vi "AddAdditionalFields.vi"(8 "error in (no error)":errorcluster, 10 "Menu":refnum<class "MGI_Menu.lvclass">, 11 "MGI_TrayItem in":refnum<class "MGI_TrayItem.lvclass">) -> (0 "error out":errorcluster, 2 "Menu out":refnum<class "MGI_Menu.lvclass">, 3 "MGI_TrayItem out":refnum<class "MGI_TrayItem.lvclass">)   [LabVIEW 2016, in "MGI_TrayItem.lvclass"]
doc: "Adds shorcut and default item indicators to the menu.\n\nAuthored by Derek E. Trepanier\nsupport@mooregoodideas.com\nwww.mooregoodideas.com\n\nCopyright (c) 2012, Moore Good Ideas, Inc.\n\nAll rights reserved.\n\nRedistribution and use in source and binary forms, with or without modification, are permitted provided that the following conditions are met:\n\n * Redistributions of source code must retain the above copyright notice, this list of conditions and the following disclaimer.\n * Redistributions in binary form must reproduce the above copyright notice, this list of conditions and the following disclaimer in the documentation and/or other materials provided with the distribution.\n * Neither the name of Moore Good Ideas, Inc. nor the names of its contributors may be used to endorse or promote products derived from this software without specific prior written permission.\n\nTHIS SOFTWARE IS PROVIDED BY THE COPYRIGHT HOLDERS AND CONTRIBUTORS \"AS IS\" AND ANY EXPRESS OR IMPLIED WARRANTIES, INCLUDING, BUT NOT LIMITED TO, THE IMPLIED WARRANTIES OF MERCHANTABILITY AND FITNESS FOR A PARTICULAR PURPOSE ARE DISCLAIMED. IN NO EVENT SHALL THE COPYRIGHT OWNER OR CONTRIBUTORS BE LIABLE FOR ANY DIRECT, INDIRECT, INCIDENTAL, SPECIAL, EXEMPLARY, OR CONSEQUENTIAL DAMAGES (INCLUDING, BUT NOT LIMITED TO, PROCUREMENT OF SUBSTITUTE GOODS OR SERVICES; LOSS OF USE, DATA, OR PROFITS; OR BUSINESS INTERRUPTION) HOWEVER CAUSED AND ON ANY THEORY OF LIABILITY, WHETHER IN CONTRACT, STRICT LIABILITY, OR TORT (INCLUDING NEGLIGENCE OR OTHERWISE) ARISING IN ANY WAY OUT OF THE USE OF THIS SOFTWARE, EVEN IF ADVISED OF THE POSSIBILITY OF SUCH DAMAGE."
uses:
  <userlib>/_MGI/Menu Building/MenuItem/TrayIcon/MGI_TrayItem.lvclass
  C:/Program Files (x86)/National Instruments/LabVIEW 2016/user.lib/_MGI/Menu Building/MenuItem/MGI_MenuItem.lvclass
  <userlib>/_MGI/Menu Building/MenuTypes/MGI_Menu.lvclass
  <userlib>/_MGI/Menu Building/MenuTypes/TrayIcon/MGI_TrayIcon.lvclass
  C:/Program Files (x86)/National Instruments/LabVIEW 2016/user.lib/_MGI/Menu Building/MenuTypes/MGI_Menu.lvclass
  <userlib>/_MGI/Menu Building/MenuItem/TrayIcon/MGI_TrayItem.lvclass/MGI_TrayItem.ctl
  System.Windows.Forms
  <userlib>/_MGI/Menu Building/MenuItem/Read Full Tag.vi
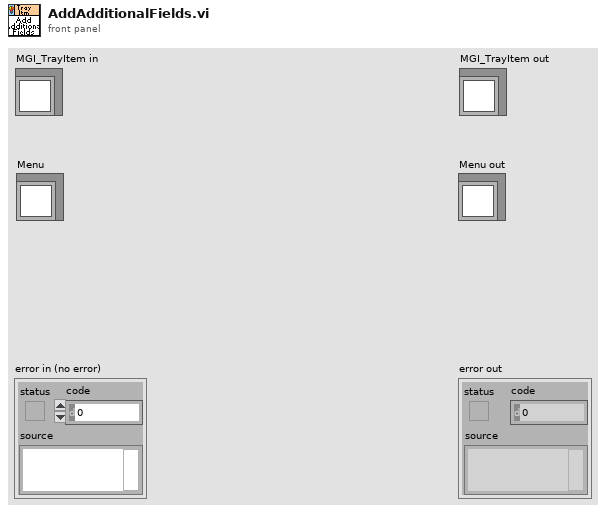
[diagram p1: front panel]
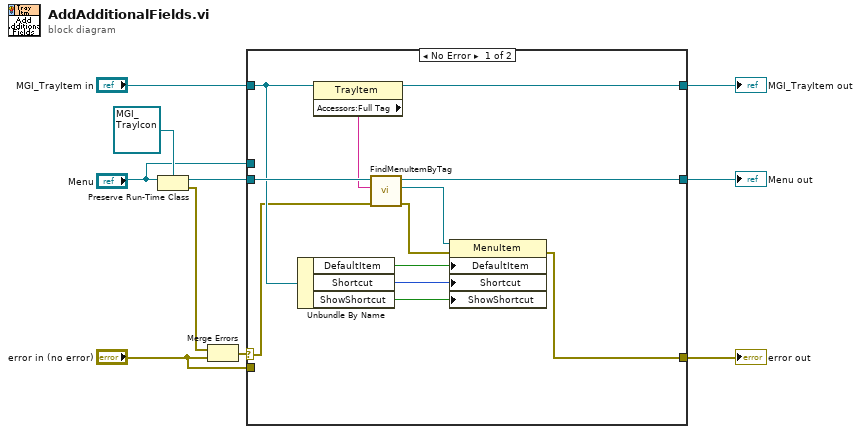
[diagram p0: block diagram]
diagram:
  n1 = Preserve Run-Time Class(object in="Menu", 2:refnum<class "MGI_TrayIcon.lvclass"> refnum ("NotifyIcon.lvclass")) -> (object out=w3:refnum<class "MGI_TrayIcon.lvclass">, error out=w8:errorcluster)  [unwired: 1 in]
  n2 = Merge Errors(w8, "error in (no error)") -> (w9:errorcluster)
  n3 = case shown="No Error" w9 {
    selector: w9 -> [w11 _]
    tunnel: [w19 w25] -> w7
    tunnel: "MGI_TrayItem in" -> [w17 w25]
    tunnel: [w20 w24] -> w5
    tunnel: "Menu" -> [_ w24]
    tunnel: w3 -> [w22 _]
    tunnel: [w12 w23] -> w2
    tunnel: "error in (no error)" -> [_ w23]
    frame No Error {
      n4 = Unbundle By Name(w17) -> ("DefaultItem"=w16:bool, "Shortcut"=w14:i32, "ShowShortcut"=w15:bool)
      n5 = property class="TrayItem"(reference=w17) -> (reference out=w19:refnum<class "MGI_TrayItem.lvclass">, "Accessors:Full Tag"=w21:string)  [unwired: 1 in, 1 out]
      n6 = call <userlib>:"FindMenuItemByTag.vi"("error in (no error)"=w11, "Full Tag"=w21, "NotifyIcon in"=w22) -> ("error out"=w13:errorcluster, "Menu Item"=w18:refnum<k24>, "NotifyIcon out"=w20:refnum<class "MGI_TrayIcon.lvclass">)  [unwired: 6 in]
      n7 = property class="MenuItem"(reference=w18, error in=w13, "DefaultItem"=w16, "Shortcut"=w14, "ShowShortcut"=w15) -> (error out=w12:errorcluster)  [unwired: 1 out]
    }
    frame Error {
      # "I dont want the cast error to propogate, but i do want it\nto cause a no-op"
    }
  }
  "error out" <- w2
  "MGI_TrayItem out" <- w7
  "Menu out" <- w5
